vi "Core gRPC Server.vi"(8 "error in (no error)":errorcluster, 11 "CIFTemplateNode in":refnum<class "CIFCorePlugin.lvclass">) -> (0 "error out":errorcluster, 3 "CIFTemplateNode out":refnum<class "CIFCorePlugin.lvclass">)   [LabVIEW 2021, in "CIFCorePlugin.lvclass"]
uses:
  CIFCorePlugin.lvclass
  CIFCoreGrpc/CIFCorePlugin_server/RPC Service/PluginCore/PluginCore.lvclass
  CIFCorePlugin.lvclass/CIFCorePlugin.ctl
  CIFCoreGrpc/CIFCorePlugin_server/RPC Service/PluginCore/PluginCore.lvclass/PluginCore.ctl
  CIFCoreGrpc/CIFCorePlugin_server/RPC Messages/cif_plugincore_Status.ctl
  CIFUtilities/CIFOutOfBand/CIFOutOfBand.lvclass/CIFOutOfBand.ctl
  CIFUtilities/CIFClocks/Typedef/Errors.ctl
  CIFCoreGrpc/CIFCorePlugin_server/RPC Messages/cif_plugincore_Version.ctl
  CIFCoreGrpc/CIFCorePlugin_server/RPC Messages/cif_plugincore_Configuration.ctl
  CIFCoreGrpc/CIFCorePlugin_server/RPC Messages/cif_plugincore_PluginOverrides.ctl
  CIFCoreGrpc/CIFCorePlugin_server/RPC Messages/cif_plugincore_TimingOverrides.ctl
  Accessors/Read Status.vi
  Accessors/Read Version.vi
  CIFUtilities/CIFOutOfBand/Write OOB DVR.vi
  CIFUtilities/CIFOutOfBand/Accessors/Read Local OOB Data.vi
  CIFUtilities/CIFOutOfBand/Accessors/Write Local OOB Data.vi
  CIFUtilities/CIFOutOfBand/Utilities/Command to Bitwise Command.vi
  CIFCoreOOB/OOB_Rx/Receive/Read Configuration.vi
  CIFCoreOOB/OOB_Rx/Private/Read Payload.vi
  CIFCoreOOB/OOB_Rx/CIFCoreOOB_Rx.lvclass
  D:/dev/CIF-LVCore/src/CIFUtilities/CIFOutOfBand/CIFOutOfBand.lvclass
  <vilib>/Utility/LVClass/Get LV Class Name.vi
  <vilib>/addons/_JKI.lib/Serialization/JSON/Library/Unflatten From JSON String.vi
  CIFCoreGrpc/CIFCorePlugin_server/CIFCorePlugin_server.lvlib
  CIFCoreCommon/CIFCoreCommon.lvlib
  <vilib>/addons/_JKI.lib/Serialization/JSON/JKI JSON Serialization.lvlib
  <vilib>/gRPC/LabVIEW gRPC Servicer/Servicer/Servicer.lvclass
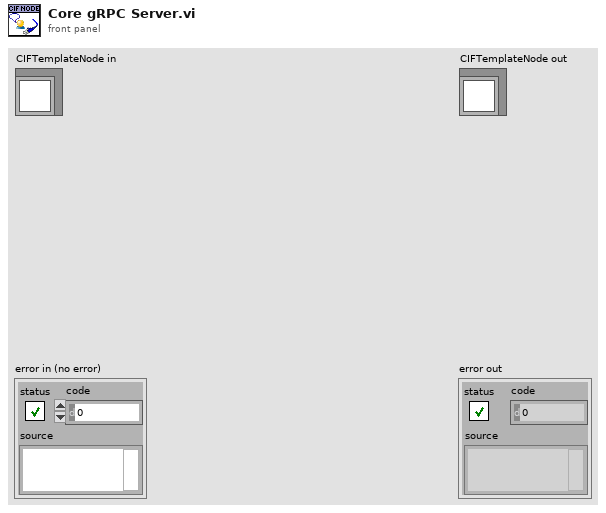
[diagram p1: front panel]
types:
  T1 = typedef "CIFCorePlugin_server.lvlib/cif_plugincore_Status.ctl" = cluster{"code":i32, "message":string}
  T2 = typedef "CIFCoreCommon.lvlib/Errors.ctl" = enum16{"Invalid Clock ID", "Long Sleep", "gRPC Server Not Found", "Config Parse", "Timestamp Wrap", "Delayed Execution"}
  T3 = typedef "CIFCorePlugin_server.lvlib/cif_plugincore_Version.ctl" = cluster{"major":u32, "minor":u32, "fix":u32, "build":u32}
  T4 = typedef "CIFCorePlugin_server.lvlib/cif_plugincore_Configuration.ctl" = cluster{"json_config":string}
  T5 = typedef "CIFCorePlugin_server.lvlib/cif_plugincore_PluginOverrides.ctl" = cluster{"timing_overrides":T6}
  T6 = typedef "CIFCorePlugin_server.lvlib/cif_plugincore_TimingOverrides.ctl" = cluster{"override_timing":bool, "period":dbl}
  T7 = typedef "CIFCorePlugin_server.lvlib/PluginCore.lvclass/Server gRPC UEs.ctl" = cluster{"PluginCore Start gRPC UE":refnum<user-event>, "PluginCore Pause gRPC UE":refnum<user-event>, "PluginCore Stop gRPC UE":refnum<user-event>, "PluginCore RefreshStatistics gRPC UE":refnum<user-event>, "PluginCore UpdateConfig gRPC UE":refnum<user-event>, "PluginCore GetStatusData gRPC UE":refnum<user-event>, "PluginCore GetVersion gRPC UE":refnum<user-event>, "PluginCore GetConfig gRPC UE":refnum<user-event>, "PluginCore GetOverrides gRPC UE":refnum<user-event>}
  T8 = typedef "grpc-lvsupport-release.lvlib/grpcId.ctl" = u64
  T9 = typedef "CIFCorePlugin_server.lvlib/cif_plugincore_FutureTimeEvent.ctl" = cluster{"fte_ns":u64}
  T10 = typedef "CIFCoreCommon.lvlib/Plugin Status.ctl" = cluster{"State":T11, "Timing Statistics (us)":T12, "FIFO Statistics (us)":T14, "error":T15, "Monitor Doubles":T16, "Monitor U64":T17, "Monitor I64":T18, "Cleanup":T13, "Create":i32, "Destroy":i32}
  T11 = typedef "CIFCoreCommon.lvlib/Plugin State.ctl" = enum32{"Null", "Creating", "Listening", "Running", "CleaningUp", "Destroying"}
  T12 = typedef "CIFCoreCommon.lvlib/Timing Statistics.ctl" = cluster{"Period":T13, "Wake Error":T13, "Execute":T13, "Housekeep":T13, "Idle":T13}
  T13 = typedef "CIFCoreCommon.lvlib/Timing Stats Base.ctl" = cluster{"Max":i32, "Min":i32}
  T14 = typedef "CIFCoreCommon.lvlib/FIFO Statistics.ctl" = cluster{"From T0":T13, "From Previous Plugin":T13, "Output Error":T13}
  T15 = typedef "CIFCoreCommon.lvlib/Simple Error.ctl" = cluster{"status":bool, "code":i32}
  T16 = typedef "CIFCoreCommon.lvlib/Monitor Doubles.ctl" = cluster{"1":dbl, "2":dbl, "3":dbl, "4":dbl}
  T17 = typedef "CIFCoreCommon.lvlib/Monitor U64.ctl" = cluster{"1":u64, "2":u64, "3":u64, "4":u64}
  T18 = typedef "CIFCoreCommon.lvlib/Monitor I64.ctl" = cluster{"1":i64, "2":i64, "3":i64, "4":i64}
  T19 = typedef "CIFCorePlugin_client.lvlib/cif_plugincore_StatusData.ctl" = cluster{"state":T20, "timing_statistics":T21, "fifo_statistics":T23, "error":T24, "monitor_doubles":T25, "monitor_u64s":T26, "monitor_i64s":T27}
  T20 = typedef "CIFCorePlugin_client.lvlib/cif_plugincore_StatusData_State.ctl" = enum32{"NULL", "CREATING", "LISTENING", "RUNNING", "CLEANINGUP", "DESTROYING"}
  T21 = typedef "CIFCorePlugin_client.lvlib/cif_plugincore_TimingStatistics.ctl" = cluster{"period":T22, "wake_error":T22, "execute":T22, "housekeep":T22, "idle":T22}
  T22 = typedef "CIFCorePlugin_client.lvlib/cif_plugincore_TimingStatsBasic.ctl" = cluster{"max":i32, "min":i32}
  T23 = typedef "CIFCorePlugin_client.lvlib/cif_plugincore_FifoStatistics.ctl" = cluster{"from_t0":T22, "from_previous_plugin":T22, "output_error":T22}
  T24 = typedef "CIFCorePlugin_client.lvlib/cif_plugincore_Error.ctl" = cluster{"status":bool, "code":i32}
  T25 = typedef "CIFCorePlugin_client.lvlib/cif_plugincore_MonitorDoubles.ctl" = cluster{"double_1":dbl, "double_2":dbl, "double_3":dbl, "double_4":dbl}
  T26 = typedef "CIFCorePlugin_client.lvlib/cif_plugincore_MonitorU64.ctl" = cluster{"u64_1":u64, "u64_2":u64, "u64_3":u64, "u64_4":u64}
  T27 = typedef "CIFCorePlugin_client.lvlib/cif_plugincore_MonitorI64.ctl" = cluster{"i64_1":i64, "i64_2":i64, "i64_3":i64, "i64_4":i64}
  T28 = typedef "CIFCoreCommon.lvlib/Version.ctl" = cluster{"Major":i32, "Minor":i32, "Fix":i32, "Build":i32}
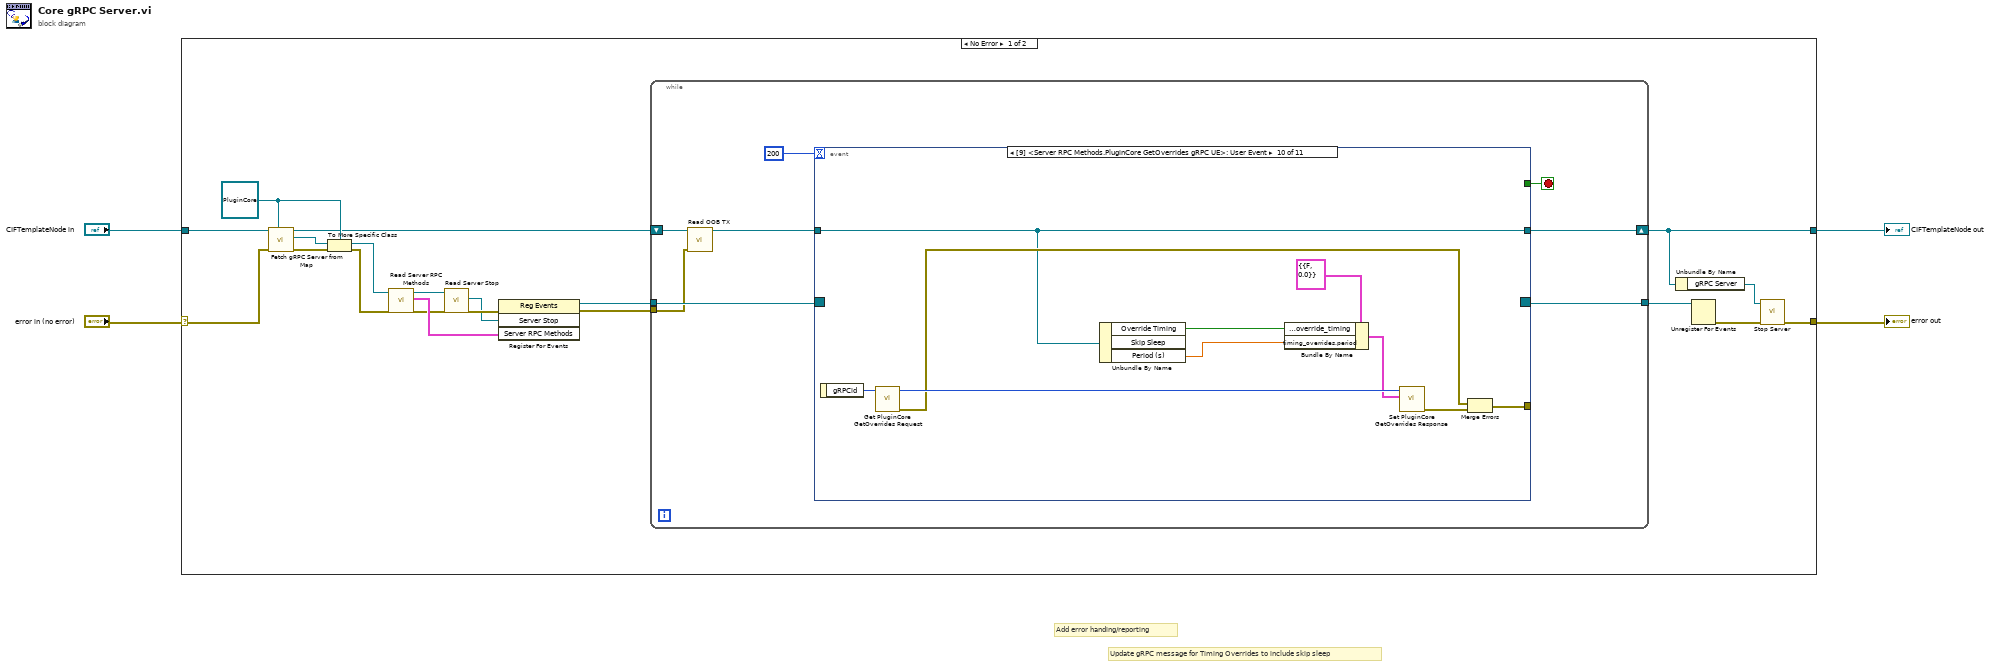
[diagram p0: block diagram]
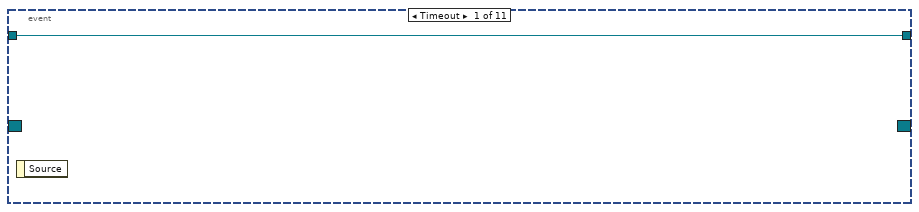
[diagram p2: hidden frame]
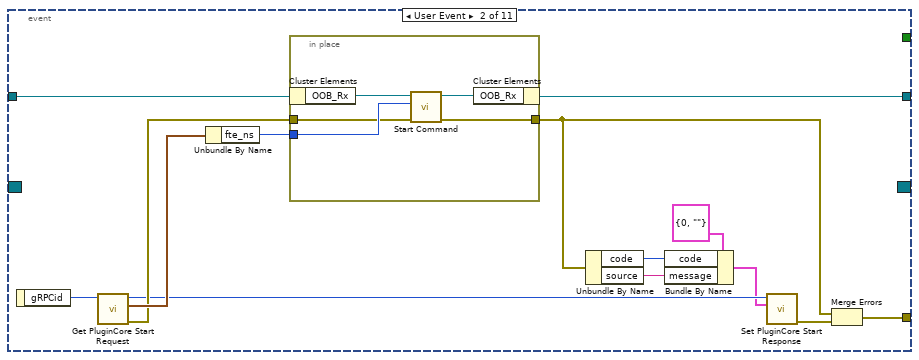
[diagram p3: hidden frame]
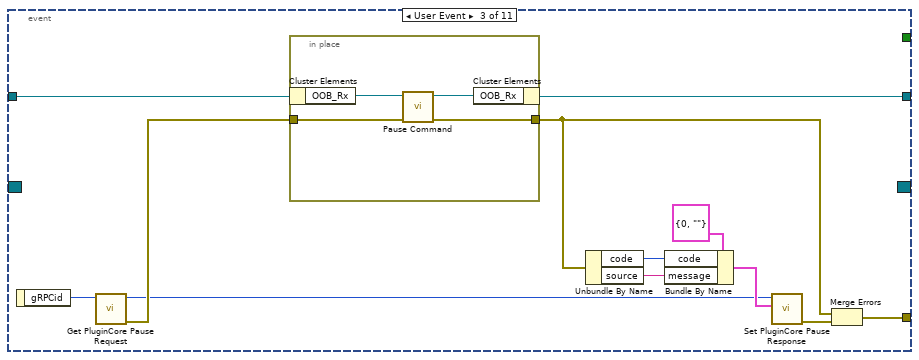
[diagram p4: hidden frame]
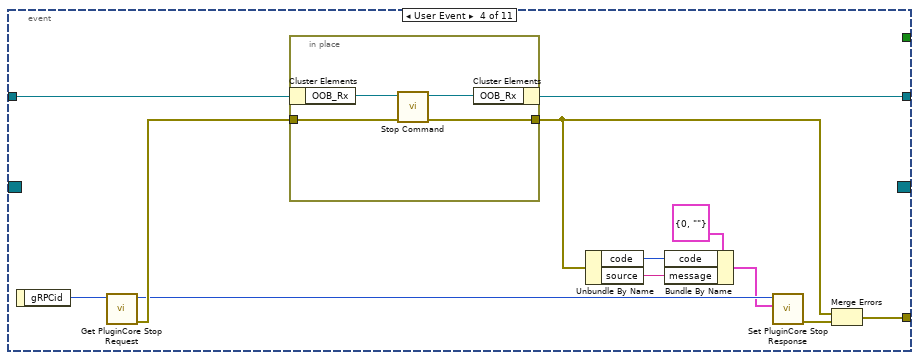
[diagram p5: hidden frame]
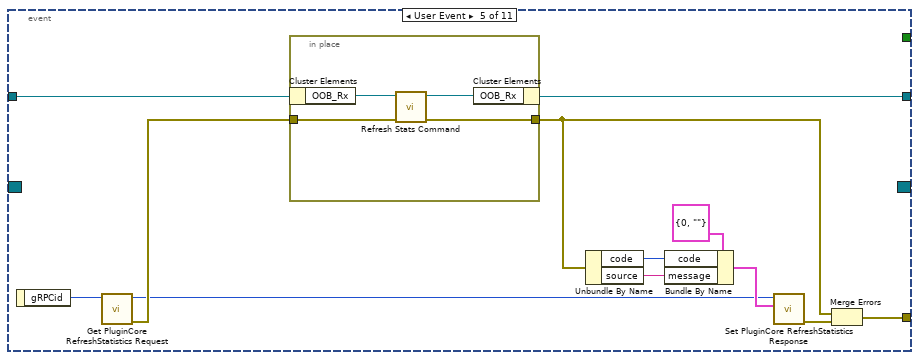
[diagram p6: hidden frame]
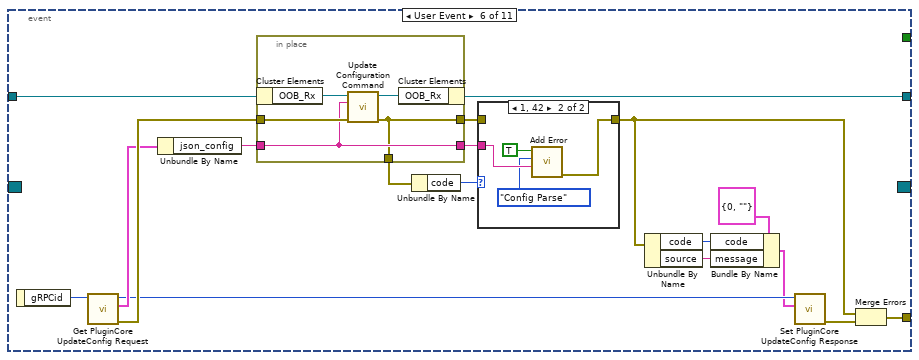
[diagram p7: hidden frame]
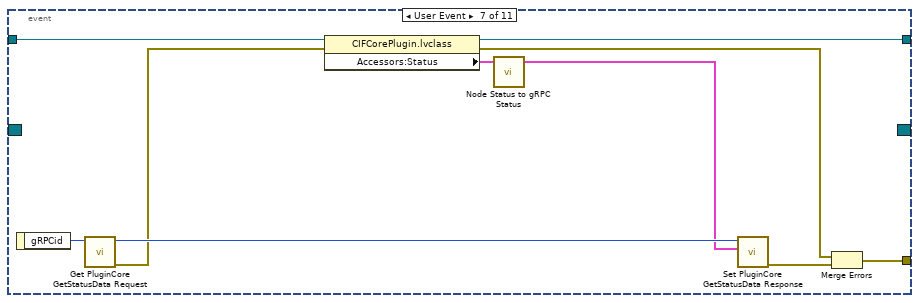
[diagram p9: hidden frame]
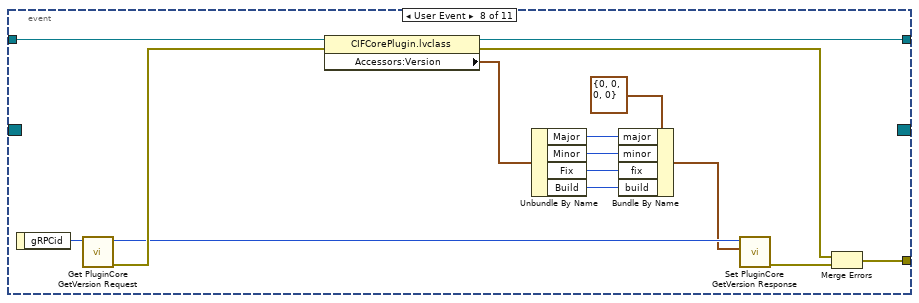
[diagram p10: hidden frame]
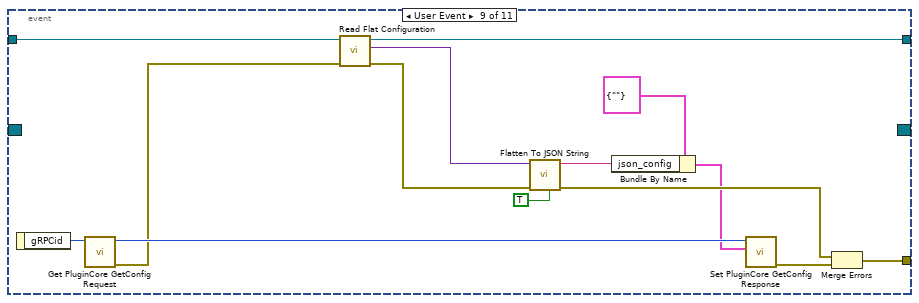
[diagram p11: hidden frame]
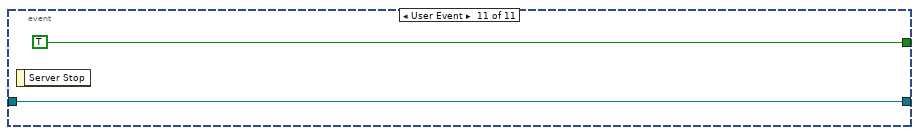
[diagram p12: hidden frame]
diagram:
  # "Update gRPC message for Timing Overrides to include skip sleep"
  # "Add error handing/reporting"
  n1 = case shown="No Error" "error in (no error)" {
    selector: "error in (no error)" -> [w23 w180]
    tunnel: "CIFTemplateNode in" -> [w24 w181]
    tunnel: [w8 w181] -> w2
    tunnel: [w5 w180] -> w1
    frame No Error {
      w20 = refnum<class "PluginCore.lvclass"> refnum ("CIFCorePlugin_server.lvlib:PluginCore.lvclass")
      n2 = call "Fetch gRPC Server from Map.vi"("gRPC Server Class type"=w20, "error in (no error)"=w23, "CIFCorePlugin in"=w24) -> ("error out"=w21:errorcluster, "gRPC Server Class out"=w22:refnum<class "PluginCore.lvclass">, "CIFCorePlugin out"=w10:refnum<class "CIFCorePlugin.lvclass">)  [unwired: 6 in]
      n3 = To More Specific Class(target class=w20, reference=w22, error in=w21) -> (specific class reference=w19:refnum<class "PluginCore.lvclass">, error out=w17:errorcluster)
      n4 = call "Read Server RPC Methods.vi"("error in (no error)"=w17, "SignalGeneratorService in"=w19) -> ("error out"=w16:errorcluster, "Server RPC Methods"=w18:T7, "SignalGeneratorService out"=w15:refnum<class "PluginCore.lvclass">)  [unwired: 7 in]
      n5 = call-dynamic "Read Server Stop.vi"("error in"=w16, "iService in"=w15) -> ("error out"=w14:errorcluster, "Server Stop"=w13:refnum<user-event>)  [unwired: 7 in, 1 out]
      n6 = register-events(error in=w14, w13, w18) -> (reference out=w12:refnum<event-registration>, error out=w11:errorcluster)  [unwired: 1 in]
      n7 = while {
        tunnel: w12 -> [w32]
        tunnel: w11 -> [w29]
        tunnel: [w25] -> w9
        shift-right: [w27] -> w8
        shift-left: w10 -> [w30]
        stop <- w26 stop-if-true
        n8 = call "Read OOB TX.vi"("error in (no error)"=w29, "CIFCorePlugin in"=w30) -> ("CIFCorePlugin out"=w28:refnum<class "CIFCorePlugin.lvclass">)  [unwired: 8 in, 1 out]
        n9 = event shown="[9] <Server RPC Methods.PluginCore GetOverrides gRPC UE>: User Event" {
          selector: w32 -> [_ _ _ _ _ _ _ _ _ _ _]
          dyn-events: [_ _ _ _ _ _ _ _ _ _ _] -> w25
          timeout: 200 -> [_ _ _ _ _ _ _ _ _ _ _]
          tunnel: w28 -> [w33 w46 w64 w80 w96 w118 w136 w152 w163 w170 w178]
          tunnel: [_ w35 w59 w75 w91 w117 w138 w153 w167 w177 _] -> _
          tunnel: [w33 w34 w58 w74 w90 w116 w135 w151 w161 w170 w178] -> w27
          tunnel: [_ _ _ _ _ _ _ _ _ _ TRUE] -> w26
          event Timeout {
            n10 = event-data() -> ()  [unwired: 1 in, 1 out]
          }
          event User Event {
            n11 = event-data() -> ("gRPCid"=w47:T8)  [unwired: 1 in]
            n12 = call "Get PluginCore Start Request.vi"("gRPCid"=w47) -> ("error out"=w43:errorcluster, "Message Data"=w45:T9, "gRPCid out"=w42:T8)  [unwired: 8 in]
            n13 = Unbundle By Name(w45) -> ("fte_ns"=w44:u64)
            n14 = in-place {
              in-place-border: w44 -> [w51]
              in-place-border: w43 -> [w50]
              in-place-border: [w48] -> w36
              n15 = in-place-cluster #1(w46) -> ("OOB_Rx"=w52:refnum<class "CIFCoreOOB_Rx.lvclass">)
              n16 = call "Start Command.vi"("error in"=w50, "FTE"=w51, "CoreOOB_Rx in"=w52) -> ("error out"=w48:errorcluster, "CoreOOB_Rx out"=w49:refnum<class "CIFCoreOOB_Rx.lvclass">)  [unwired: 7 in]
              n17 = in-place-cluster #1("OOB_Rx"=w49) -> (w34:refnum<class "CIFCorePlugin.lvclass">)
            }
            n18 = Unbundle By Name(w36) -> ("code"=w40:i32, "source"=w39:string)
            n19 = Bundle By Name(cluster=T1 {"code"=0, "message"=""} ("Message Data"), "code"=w40, "message"=w39) -> (w38:T1)
            n20 = call "Set PluginCore Start Response.vi"("Message Data"=w38, "gRPCid in"=w42) -> ("error out"=w37:errorcluster)  [unwired: 9 in]
            n21 = Merge Errors(w36, w37) -> (w35:errorcluster)
          }
          event User Event {
            n22 = event-data() -> ("gRPCid"=w57:T8)  [unwired: 1 in]
            n23 = call "Get PluginCore Pause Request.vi"("gRPCid"=w57) -> ("error out"=w56:errorcluster, "gRPCid out"=w54:T8)  [unwired: 8 in, 1 out]
            n24 = in-place {
              in-place-border: w56 -> [w66]
              in-place-border: [w65] -> w60
              n25 = in-place-cluster #2(w64) -> ("OOB_Rx"=w68:refnum<class "CIFCoreOOB_Rx.lvclass">)
              n26 = call "Pause Command.vi"("error in"=w66, "CoreOOB_Rx in"=w68) -> ("error out"=w65:errorcluster, "CoreOOB_Rx out"=w67:refnum<class "CIFCoreOOB_Rx.lvclass">)  [unwired: 8 in]
              n27 = in-place-cluster #2("OOB_Rx"=w67) -> (w58:refnum<class "CIFCorePlugin.lvclass">)
            }
            n28 = Unbundle By Name(w60) -> ("code"=w62:i32, "source"=w61:string)
            n29 = Bundle By Name(cluster=T1 {"code"=0, "message"=""} ("Message Data"), "code"=w62, "message"=w61) -> (w55:T1)
            n30 = call "Set PluginCore Pause Response.vi"("Message Data"=w55, "gRPCid in"=w54) -> ("error out"=w53:errorcluster)  [unwired: 9 in]
            n31 = Merge Errors(w60, w53) -> (w59:errorcluster)
          }
          event User Event {
            n32 = event-data() -> ("gRPCid"=w73:T8)  [unwired: 1 in]
            n33 = call "Get PluginCore Stop Request.vi"("gRPCid"=w73) -> ("error out"=w72:errorcluster, "gRPCid out"=w71:T8)  [unwired: 8 in, 1 out]
            n34 = in-place {
              in-place-border: w72 -> [w83]
              in-place-border: [w81] -> w76
              n35 = in-place-cluster #3(w80) -> ("OOB_Rx"=w84:refnum<class "CIFCoreOOB_Rx.lvclass">)
              n36 = call "Stop Command.vi"("error in"=w83, "CoreOOB_Rx in"=w84) -> ("error out"=w81:errorcluster, "CoreOOB_Rx out"=w82:refnum<class "CIFCoreOOB_Rx.lvclass">)  [unwired: 8 in]
              n37 = in-place-cluster #3("OOB_Rx"=w82) -> (w74:refnum<class "CIFCorePlugin.lvclass">)
            }
            n38 = Unbundle By Name(w76) -> ("code"=w78:i32, "source"=w77:string)
            n39 = Bundle By Name(cluster=T1 {"code"=0, "message"=""} ("Message Data"), "code"=w78, "message"=w77) -> (w70:T1)
            n40 = call "Set PluginCore Stop Response.vi"("Message Data"=w70, "gRPCid in"=w71) -> ("error out"=w69:errorcluster)  [unwired: 9 in]
            n41 = Merge Errors(w76, w69) -> (w75:errorcluster)
          }
          event User Event {
            n42 = event-data() -> ("gRPCid"=w89:T8)  [unwired: 1 in]
            n43 = call "Get PluginCore RefreshStatistics Request.vi"("gRPCid"=w89) -> ("error out"=w88:errorcluster, "gRPCid out"=w85:T8)  [unwired: 8 in, 1 out]
            n44 = in-place {
              in-place-border: w88 -> [w99]
              in-place-border: [w98] -> w92
              n45 = in-place-cluster #4(w96) -> ("OOB_Rx"=w100:refnum<class "CIFCoreOOB_Rx.lvclass">)
              n46 = call "Refresh Stats Command.vi"("error in"=w99, "CoreOOB_Rx in"=w100) -> ("error out"=w98:errorcluster, "CoreOOB_Rx out"=w97:refnum<class "CIFCoreOOB_Rx.lvclass">)  [unwired: 8 in]
              n47 = in-place-cluster #4("OOB_Rx"=w97) -> (w90:refnum<class "CIFCorePlugin.lvclass">)
            }
            n48 = Unbundle By Name(w92) -> ("code"=w94:i32, "source"=w93:string)
            n49 = Bundle By Name(cluster=T1 {"code"=0, "message"=""} ("Message Data"), "code"=w94, "message"=w93) -> (w87:T1)
            n50 = call "Set PluginCore RefreshStatistics Response.vi"("Message Data"=w87, "gRPCid in"=w85) -> ("error out"=w86:errorcluster)  [unwired: 9 in]
            n51 = Merge Errors(w92, w86) -> (w91:errorcluster)
          }
          event User Event {
            n52 = event-data() -> ("gRPCid"=w115:T8)  [unwired: 1 in]
            n53 = call "Get PluginCore UpdateConfig Request.vi"("gRPCid"=w115) -> ("error out"=w114:errorcluster, "Message Data"=w113:T4, "gRPCid out"=w110:T8)  [unwired: 8 in]
            n54 = Unbundle By Name(w113) -> ("json_config"=w112:string)
            n55 = in-place {
              in-place-border: w114 -> [w126]
              in-place-border: [w124] -> w106
              in-place-border: w112 -> [w125]
              in-place-border: [w125] -> w108
              in-place-border: [w124] -> w107
              n56 = in-place-cluster #5(w118) -> ("OOB_Rx"=w128:refnum<class "CIFCoreOOB_Rx.lvclass">)
              n57 = call "Update Configuration Command.vi"("error in"=w126, "Config JSON"=w125, "CoreOOB_Rx in"=w128) -> ("error out"=w124:errorcluster, "CoreOOB_Rx out"=w127:refnum<class "CIFCoreOOB_Rx.lvclass">)  [unwired: 7 in]
              n58 = in-place-cluster #5("OOB_Rx"=w127) -> (w116:refnum<class "CIFCorePlugin.lvclass">)
            }
            n59 = Unbundle By Name(w107) -> ("code"=w109:i32)
            n60 = case shown="1, 42" w109 {
              tunnel: w106 -> [w119 _]
              tunnel: [w119 w123] -> w101
              tunnel: w108 -> [_ w122]
              frame 0, Default {
              }
              frame 1, 42 {
                n61 = call "Add Error.vi"("String to Append"=w122, "Error"=Errors."Config Parse", "Insert Error"=TRUE) -> ("error out"=w123:errorcluster)  [unwired: 8 in]
              }
            }
            n62 = Unbundle By Name(w101) -> ("code"=w105:i32, "source"=w104:string)
            n63 = Bundle By Name(cluster=T1 {"code"=0, "message"=""} ("Message Data"), "code"=w105, "message"=w104) -> (w102:T1)
            n64 = call "Set PluginCore UpdateConfig Response.vi"("Message Data"=w102, "gRPCid in"=w110) -> ("error out"=w111:errorcluster)  [unwired: 9 in]
            n65 = Merge Errors(w101, w111) -> (w117:errorcluster)
          }
          event User Event {
            n66 = event-data() -> ("gRPCid"=w137:T8)  [unwired: 1 in]
            n67 = call "Get PluginCore GetStatusData Request.vi"("gRPCid"=w137) -> ("error out"=w130:errorcluster, "gRPCid out"=w132:T8)  [unwired: 8 in, 1 out]
            n68 = property class="CIFCorePlugin.lvclass"(reference=w136, error in=w130) -> (reference out=w135:refnum<class "CIFCorePlugin.lvclass">, error out=w129:errorcluster, "Accessors:Status"=w134:T10)
            n69 = call "Node Status to gRPC Status.vi"("Node Status"=w134) -> ("gRPC Status"=w131:T19)  [unwired: 3 in]
            n70 = call "Set PluginCore GetStatusData Response.vi"("Message Data"=w131, "gRPCid in"=w132) -> ("error out"=w133:errorcluster)  [unwired: 9 in]
            n71 = Merge Errors(w129, w133) -> (w138:errorcluster)
          }
          event User Event {
            n72 = event-data() -> ("gRPCid"=w149:T8)  [unwired: 1 in]
            n73 = call "Get PluginCore GetVersion Request.vi"("gRPCid"=w149) -> ("error out"=w148:errorcluster, "gRPCid out"=w147:T8)  [unwired: 8 in, 1 out]
            n74 = property class="CIFCorePlugin.lvclass"(reference=w152, error in=w148) -> (reference out=w151:refnum<class "CIFCorePlugin.lvclass">, error out=w150:errorcluster, "Accessors:Version"=w140:T28)
            n75 = Unbundle By Name(w140) -> ("Major"=w144:i32, "Minor"=w143:i32, "Fix"=w142:i32, "Build"=w141:i32)
            n76 = Bundle By Name(cluster=T3 {"major"=0, "minor"=0, "fix"=0, "build"=0} ("Message Data"), "major"=w144, "minor"=w143, "fix"=w142, "build"=w141) -> (w139:T3)
            n77 = call "Set PluginCore GetVersion Response.vi"("Message Data"=w139, "gRPCid in"=w147) -> ("error out"=w146:errorcluster)  [unwired: 9 in]
            n78 = Merge Errors(w150, w146) -> (w153:errorcluster)
          }
          event User Event {
            n79 = event-data() -> ("gRPCid"=w166:T8)  [unwired: 1 in]
            n80 = call "Get PluginCore GetConfig Request.vi"("gRPCid"=w166) -> ("error out"=w162:errorcluster, "gRPCid out"=w165:T8)  [unwired: 8 in, 1 out]
            n81 = call "Read Flat Configuration.vi"("error in (no error)"=w162, "CIFTemplateNode in"=w163) -> ("error out"=w159:errorcluster, "Configuration"=w160:variant, "CIFTemplateNode out"=w161:refnum<class "CIFCorePlugin.lvclass">)  [unwired: 7 in]
            n82 = call <vilib>:"Flatten To JSON String.vi"("Enums As String (F)"=TRUE, "error in (no error)"=w159, "Variant"=w160) -> ("error out"=w157:errorcluster, "JSON String"=w156:string)  [unwired: 7 in]
            n83 = Bundle By Name(cluster=T4 {"json_config"=""} ("Message Data"), "json_config"=w156) -> (w155:T4)
            n84 = call "Set PluginCore GetConfig Response.vi"("Message Data"=w155, "gRPCid in"=w165) -> ("error out"=w164:errorcluster)  [unwired: 9 in]
            n85 = Merge Errors(w157, w164) -> (w167:errorcluster)
          }
          event User Event {
            n86 = event-data() -> ("gRPCid"=w176:T8)  [unwired: 1 in]
            n87 = call "Get PluginCore GetOverrides Request.vi"("gRPCid"=w176) -> ("error out"=w171:errorcluster, "gRPCid out"=w175:T8)  [unwired: 8 in, 1 out]
            n88 = Unbundle By Name(w170) -> ("Override Timing"=w169:bool, "Period (s)"=w168:dbl)  [unwired: 1 out]
            n89 = Bundle By Name(cluster=T5 {"timing_overrides"={"override_timing"=FALSE, "period"=0.0}} ("Message Data"), "timing_overrides.override_timing"=w169, "timing_overrides.period"=w168) -> (w172:T5)
            n90 = call "Set PluginCore GetOverrides Response.vi"("Message Data"=w172, "gRPCid in"=w175) -> ("error out"=w174:errorcluster)  [unwired: 9 in]
            n91 = Merge Errors(w171, w174) -> (w177:errorcluster)
          }
          event User Event {
            n92 = event-data() -> ()  [unwired: 1 in, 1 out]
          }
        }
      }
      n93 = Unbundle By Name(w8) -> ("gRPC Server"=w7:refnum<class "Servicer.lvclass">)
      n94 = Unregister For Events(event registration refnum=w9) -> (error out=w6:errorcluster)  [unwired: 1 in]
      n95 = call <vilib>:"Stop Server.vi"("error in"=w6, "gRPC Server in"=w7) -> ("error out"=w5:errorcluster)  [unwired: 9 in]
    }
    frame Error {
    }
  }
  "error out" <- w1
  "CIFTemplateNode out" <- w2
